vi "Get Parent Message Class Path.vi"(8 "error in (no error)":errorcluster, 11 "Concrete Message Scripter in":refnum<class "Concrete Message Scripter.lvclass">) -> (0 "error out":errorcluster, 2 "Parent Message":path)   [LabVIEW 2020, in "Message Maker.lvlib" / "Concrete Message Scripter.lvclass"]
uses:
  Concrete Message Scripter.lvclass
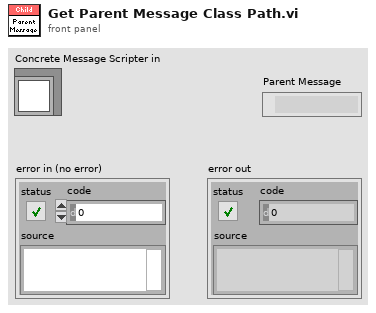
[diagram p1: front panel]
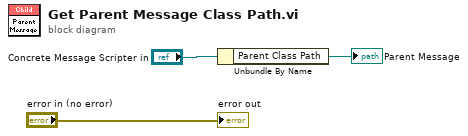
[diagram p0: block diagram]
diagram:
  n1 = Unbundle By Name("Concrete Message Scripter in") -> ("Parent Class Path"=→"Parent Message":path)
  "error out" <- "error in (no error)"
